vi "movestage_troubleshoot.vi"() -> ()   [LabVIEW 2013]
uses:
  <vilib>/Instr/_visa.llb/VISA Configure Serial Port (Instr).vi
panel:
  in  "x or y":bool
  out "error out":errorcluster
  in  "stage_move":i32
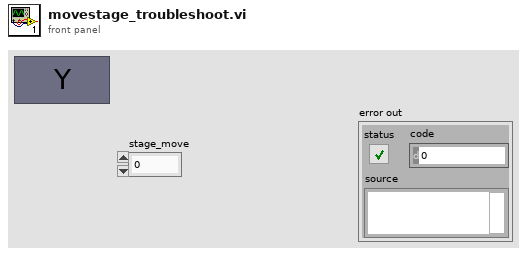
[diagram p1: front panel]
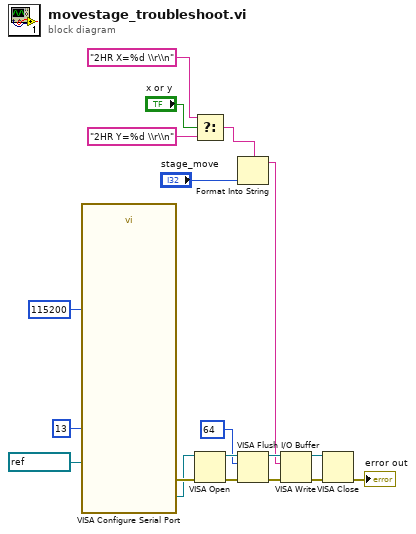
[diagram p0: block diagram]
diagram:
  n1 = call-poly "VISA Configure Serial Port"("VISA resource name"=refnum<visa-resource-name> "COM1", "termination char\n(0xA = '\\n' = LF)"=u8 13 ("termination char\n(0xA = '\\n' = LF)"), "baud rate (9600)"=u32 115200 ("baud rate (9600) 2")) -> ("VISA resource name out"=w14:refnum<visa-resource-name>, "error out"=w18:errorcluster)  [unwired: 4 in, 7 out]
  n2 = Select(t="2HR X=%d \\r\\n" ("format string"), s="x or y", f="2HR Y=%d \\r\\n" ("format string")) -> (s? t:f=w1:string)
  n3 = VISA Open(error in (no error)=w18, VISA resource name=w14) -> (VISA resource name=w15:refnum<visa-resource-name>, error out=w19:errorcluster)  [unwired: 3 in]
  n4 = Format Into String(format string=w1, "stage_move") -> (resulting string=w9:string)  [unwired: 2 in, 1 out]
  n5 = VISA Flush I/O Buffer(VISA resource name=w15, mask (16)=u16 64, error in (no error)=w19) -> (VISA resource name out=w10:refnum<visa-resource-name>, error out=w11:errorcluster)
  n6 = VISA Write(VISA resource name=w10, write buffer=w9, error in (no error)=w11) -> (VISA resource name out=w16:refnum<visa-resource-name>, error out=w17:errorcluster)  [unwired: 1 out]
  n7 = VISA Close(VISA resource name=w16, error in (no error)=w17) -> (error out=→"error out":errorcluster)
